vi "Pre Launch Init.vi"(11 "Nested in":refnum<class "UI Actor.lvclass">) -> (0 "error out":errorcluster, 3 "Nested out":refnum<class "UI Actor.lvclass">)   [LabVIEW 2019, in "UI Actor.lvlib" / "UI Actor.lvclass"]
doc: "(<B>Filename</B>: Actor Framework.lvlib:Actor.lvclass:Pre Launch Init.vi)\n\nDefines behavior that occurs after the Launch Nested Actor method is invoked but before the actor's Actor Core method begins running.\n\nBy default, this method does nothing. A descendant class may override it to define behavior."
uses:
  UI Actor.lvclass
  C:/Program Files (x86)/National Instruments/LabVIEW 2019/vi.lib/ActorFramework/Actor/Actor.lvclass
  UI Actor.lvclass/UI Actor.ctl
  <vilib>/ActorFramework/Actor/Actor.lvclass/Actor.ctl
  <vilib>/ActorFramework/Message Enqueuer/Message Enqueuer.lvclass/Message Enqueuer.ctl
  <vilib>/ActorFramework/Message Enqueuer/Init from Existing Queue.vi
  <vilib>/ActorFramework/Message Enqueuer/Enqueue.vi
  UI Actor Messages/INIT Msg/INIT Msg.lvclass
  C:/Program Files (x86)/National Instruments/LabVIEW 2019/vi.lib/ActorFramework/Message/Message.lvclass
  <vilib>/ActorFramework/Message Priority Queue/Priority Enqueue.vi
  <vilib>/ActorFramework/Message Enqueuer/Message Enqueuer.lvclass
  <vilib>/ActorFramework/Actor/Actor.lvclass
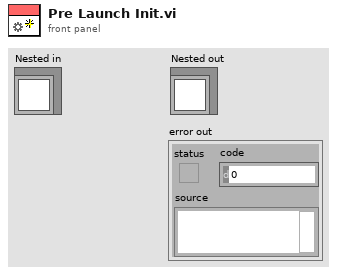
[diagram p1: front panel]
types:
  T1 = cluster{"Inventario":i32, "Producto":string, "Costo":dbl}
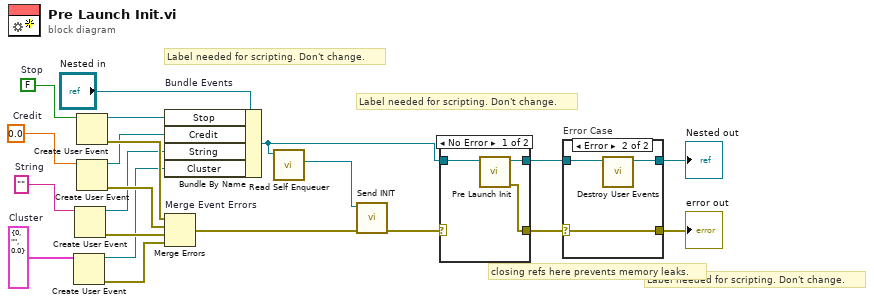
[diagram p0: block diagram]
diagram:
  w3 = T1 {"Inventario"=0, "Producto"="", "Costo"=0.0}  # Cluster
  w6 = ""  # String
  w9 = 0.0  # Credit
  w20 = FALSE  # Stop
  # "Label needed for scripting. Don't change."
  # "Label needed for scripting. Don't change."
  # "Label needed for scripting. Don't change."
  # "closing refs here prevents memory leaks."
  n1 = Create User Event(user event datatype=w3) -> (user event=w2:refnum<user-event>, error out=w1:errorcluster)  [unwired: 1 in]
  n2 = Create User Event(user event datatype=w6) -> (user event=w5:refnum<user-event>, error out=w4:errorcluster)  [unwired: 1 in]
  n3 = Create User Event(user event datatype=w20) -> (user event=w17:refnum<user-event>, error out=w19:errorcluster)  [unwired: 1 in]
  n4 = Create User Event(user event datatype=w9) -> (user event=w8:refnum<user-event>, error out=w7:errorcluster)  [unwired: 1 in]
  n5 = Bundle By Name "Bundle Events"(cluster="Nested in", "Stop"=w17, "Credit"=w8, "String"=w5, "Cluster"=w2) -> (w13:refnum<class "UI Actor.lvclass">)
  n6 = Merge Errors "Merge Event Errors"(w19, w7, w4, w1) -> (w11:errorcluster)
  n7 = call <vilib>:"Read Self Enqueuer.vi"("Actor"=w13) -> ("Self Enqueuer"=w12:refnum<class "Message Enqueuer.lvclass">)  [unwired: 10 in]
  n8 = call "Send INIT.vi"("error in (no error)"=w11, "Message Enqueuer"=w12) -> ("error out"=w10:errorcluster)  [unwired: 8 in, 1 out]
  n9 = case shown="No Error" w10 {
    selector: w10 -> [_ w26]
    tunnel: [w24 w25] -> w15
    tunnel: w13 -> [w23 w25]
    tunnel: [w22 w26] -> w14
    frame No Error {
      n10 = call-parent "Pre Launch Init.vi"("Actor in"=w23) -> ("error out"=w22:errorcluster, "Actor out"=w24:refnum<class "UI Actor.lvclass">)  [unwired: 9 in]
    }
    frame Error {
    }
  }
  n11 = case "Error Case" shown="Error" w14 {
    selector: w14 -> [w27 w31]
    tunnel: w15 -> [w28 w30]
    tunnel: [w28 w29] -> w18
    tunnel: [w27 w31] -> w16
    frame No Error {
    }
    frame Error {
      n12 = call "Destroy User Events.vi"("UI Template in"=w30) -> ("UI Template out"=w29:refnum<class "UI Actor.lvclass">)  [unwired: 10 in]
    }
  }
  "error out" <- w16
  "Nested out" <- w18
